vi "WS2812 Controller.vi"() -> ()   [LabVIEW 2017]
uses:
  IMAQCV/PIIO/Core/PIIO DIO.ctl
  IMAQCV/PIIO.lvlib
panel:
  in  "PIN":T1 items=["L1", "L2"]
  out "size(s)":i32
  in  "Number of LEDs":u16=40
  in  "Red Phase Multiplier":dbl=10.0 caption="Phase"
  in  "Red Phase Offset":dbl=10.0 caption="Phase"
  in  "Green Phase Multiplier":dbl=10.0 caption="Phase"
  in  "Green Phase Offset":dbl=10.0 caption="Phase"
  in  "Blue Phase Multiplier":dbl=10.0 caption="Phase"
  in  "Blue Phase Offset":dbl=10.0 caption="Phase"
  in  "Red Intensity Multiplier":dbl=1.0 caption="Phase" min=0.0 max=1.0
  in  "Green Intensity Multiplier":dbl=1.0 caption="Phase" min=0.0 max=1.0
  in  "Blue Intensity Multiplier":dbl=1.0 caption="Phase" min=0.0 max=1.0
  in  "Red Waveform":enum16{"Sine", "Square", "Triangle", "Sawtooth"}(ring)
  in  "Green Waveform":enum16{"Sine", "Square", "Triangle", "Sawtooth"}(ring)
  in  "Blue Waveform":enum16{"Sine", "Square", "Triangle", "Sawtooth"}(ring)
  in  "Red Duty Cycle":dbl=1.0 caption="Phase" min=0.0 max=100.0
  in  "Green Duty Cycle":dbl=1.0 caption="Phase" min=0.0 max=50.0
  in  "Blue Duty Cycle":dbl=1.0 caption="Phase" min=0.0 max=100.0
  in  "Stop Button":bool
  out "RGB Values":dynamicdata(graph)
  # "Duty Cycle\n(Square Wave)"
  # "Intensity (0-1)"
  # "Phase Multiplier"
  # "Phase Offset"
  # "Waveform"
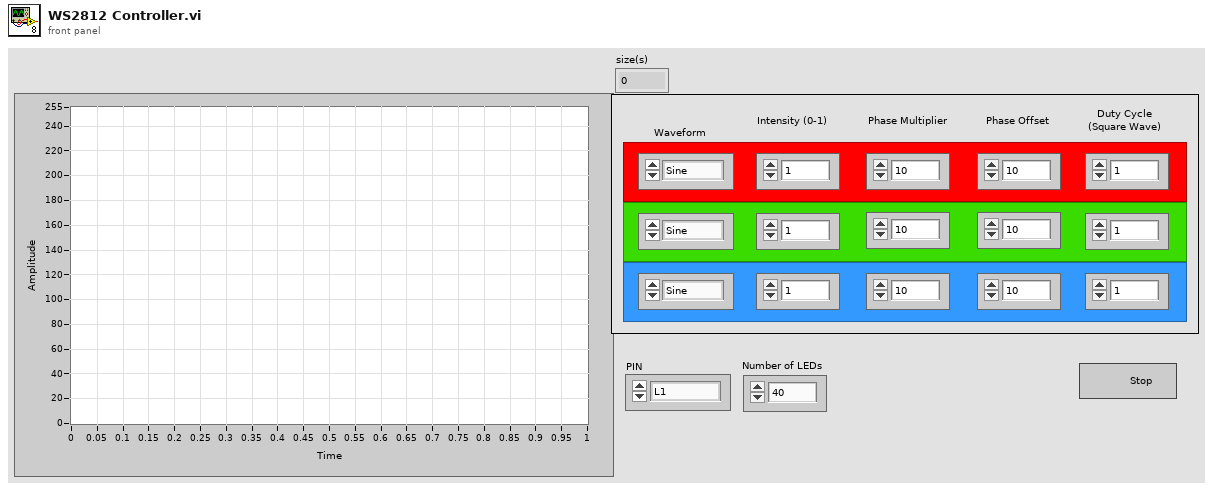
[diagram p1: front panel]
types:
  T1 = typedef "PIIO.lvlib/PIIO DIO.ctl" = u8
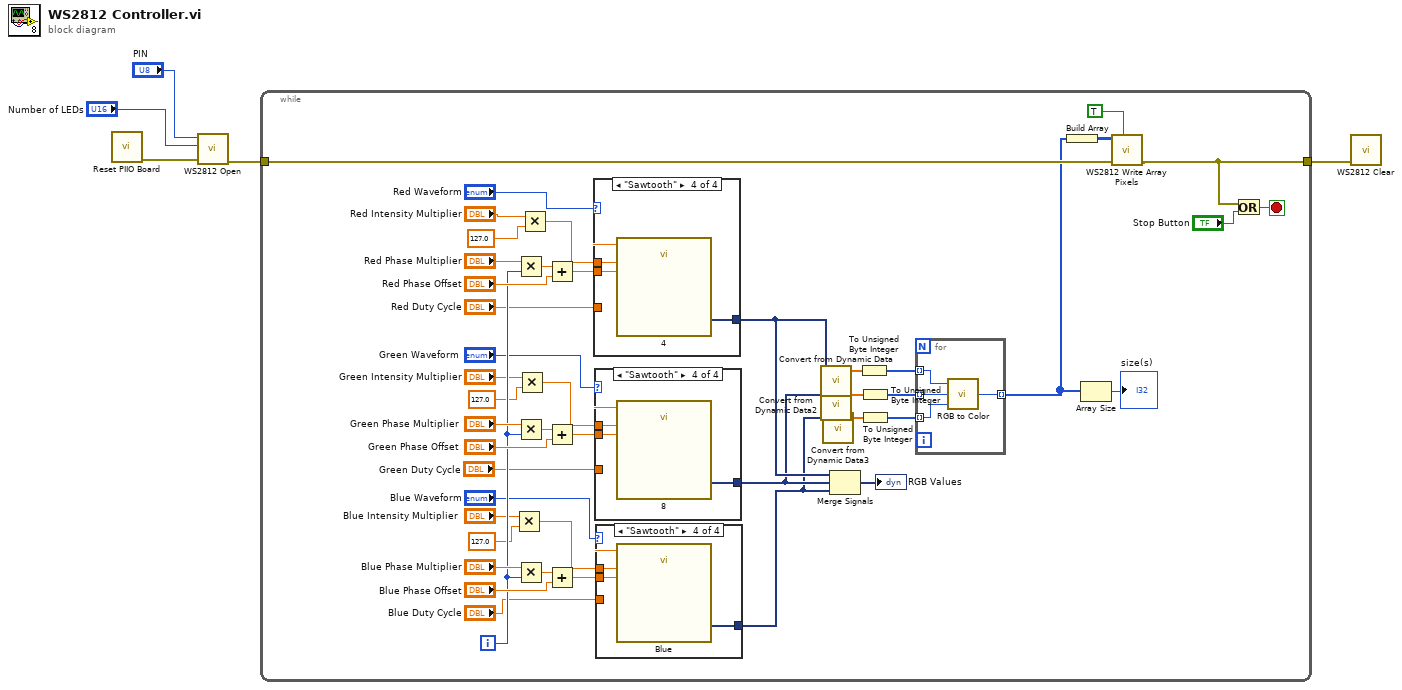
[diagram p0: block diagram]
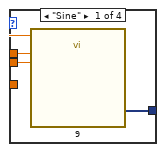
[diagram p2: hidden frame]
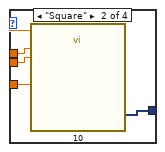
[diagram p3: hidden frame]
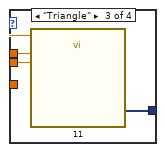
[diagram p4: hidden frame]
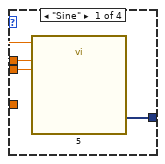
[diagram p5: hidden frame]
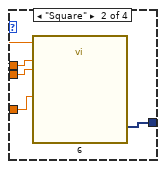
[diagram p6: hidden frame]
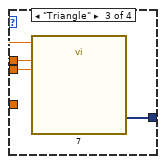
[diagram p7: hidden frame]
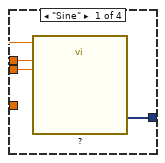
[diagram p8: hidden frame]
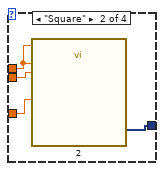
[diagram p9: hidden frame]
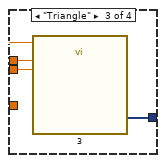
[diagram p10: hidden frame]
diagram:
  n1 = call "Reset PIIO Board.vi"() -> ("error out"=w2:errorcluster)  [unwired: 11 in]
  n2 = call "WS2812 Open.vi"("Error In"=w2, "Number of LEDs"="Number of LEDs", "PIN"="PIN") -> ("Error Out"=w5:errorcluster)  [unwired: 8 in]
  n3 = while {
    tunnel: w5 -> [w11]
    tunnel: [w10] -> w3
    i -> [w29]
    stop <- w51 stop-if-true
    n4 = Multiply(x="Blue Intensity Multiplier", y=127.0) -> (x*y=w19:dbl)
    n5 = Multiply(x="Red Phase Multiplier", y=w29) -> (x*y=w27:dbl)
    n6 = Multiply(x="Green Phase Multiplier", y=w29) -> (x*y=w45:dbl)
    n7 = Multiply(x="Blue Phase Multiplier", y=w29) -> (x*y=w42:dbl)
    n8 = Multiply(x="Green Intensity Multiplier", y=127.0) -> (x*y=w21:dbl)
    n9 = Multiply(x="Red Intensity Multiplier", y=127.0) -> (x*y=w20:dbl)
    n10 = Add(x=w27, y="Red Phase Offset") -> (x+y=w48:dbl)
    n11 = Add(x=w45, y="Green Phase Offset") -> (x+y=w47:dbl)
    n12 = Add(x=w42, y="Blue Phase Offset") -> (x+y=w40:dbl)
    n13 = case shown="\"Sawtooth\"" "Red Waveform" {
      tunnel: w48 -> [w80 w84 w87 w90]
      tunnel: [w79 w83 w86 w89] -> w33
      tunnel: w20 -> [w78 w82 w85 w88]
      tunnel: "Red Duty Cycle" -> [_ w81 _ _]
      frame "Sine" {
        n14 = call "?"("Offset"=w78, "Amplitude"=w78, "Phase"=w80) -> ("Red Sine"=w79:dynamicdata)  [unwired: 11 in, 1 out]
      }
      frame "Square" {
        n15 = call "2"("Offset"=w82, "Duty Cycle (%)"=w81, "Amplitude"=w82, "Phase"=w84) -> ("Red Square"=w83:dynamicdata)  [unwired: 10 in, 1 out]
      }
      frame "Triangle" {
        n16 = call "3"("Offset"=w85, "Amplitude"=w85, "Phase"=w87) -> ("Red Triangle"=w86:dynamicdata)  [unwired: 11 in, 1 out]
      }
      frame "Sawtooth" {
        n17 = call "4"("Offset"=w88, "Amplitude"=w88, "Phase"=w90) -> ("Red Sawtooth"=w89:dynamicdata)  [unwired: 11 in, 1 out]
      }
    }
    n18 = case shown="\"Sawtooth\"" "Green Waveform" {
      tunnel: w47 -> [w67 w71 w74 w77]
      tunnel: [w66 w70 w73 w76] -> w32
      tunnel: w21 -> [w65 w69 w72 w75]
      tunnel: "Green Duty Cycle" -> [_ w68 _ _]
      frame "Sine" {
        n19 = call "5"("Offset"=w65, "Amplitude"=w65, "Phase"=w67) -> ("Green Sine"=w66:dynamicdata)  [unwired: 11 in, 1 out]
      }
      frame "Square" {
        n20 = call "6"("Offset"=w69, "Duty Cycle (%)"=w68, "Amplitude"=w69, "Phase"=w71) -> ("Green Square"=w70:dynamicdata)  [unwired: 10 in, 1 out]
      }
      frame "Triangle" {
        n21 = call "7"("Offset"=w72, "Amplitude"=w72, "Phase"=w74) -> ("Green Triange"=w73:dynamicdata)  [unwired: 11 in, 1 out]
      }
      frame "Sawtooth" {
        n22 = call "8"("Offset"=w75, "Amplitude"=w75, "Phase"=w77) -> ("Green Sawtooth"=w76:dynamicdata)  [unwired: 11 in, 1 out]
      }
    }
    n23 = case shown="\"Sawtooth\"" "Blue Waveform" {
      tunnel: w40 -> [w54 w58 w61 w64]
      tunnel: [w53 w57 w60 w63] -> w31
      tunnel: w19 -> [w52 w56 w59 w62]
      tunnel: "Blue Duty Cycle" -> [_ w55 _ _]
      frame "Sine" {
        n24 = call "9"("Offset"=w52, "Amplitude"=w52, "Phase"=w54) -> ("Blue Sine"=w53:dynamicdata)  [unwired: 11 in, 1 out]
      }
      frame "Square" {
        n25 = call "10"("Offset"=w56, "Duty Cycle (%)"=w55, "Amplitude"=w56, "Phase"=w58) -> ("Blue Square"=w57:dynamicdata)  [unwired: 10 in, 1 out]
      }
      frame "Triangle" {
        n26 = call "11"("Offset"=w59, "Amplitude"=w59, "Phase"=w61) -> ("Blue Triangle"=w60:dynamicdata)  [unwired: 11 in, 1 out]
      }
      frame "Sawtooth" {
        n27 = call "Blue"("Offset"=w62, "Amplitude"=w62, "Phase"=w64) -> ("Blue Sawtooth"=w63:dynamicdata)  [unwired: 11 in, 1 out]
      }
    }
    n28 = call "Convert from Dynamic Data"("Dynamic Data Type"=w33) -> ("Array"=w39:dbl[])  [unwired: 3 in]
    n29 = call "Convert from Dynamic Data2"("Dynamic Data Type"=w32) -> ("Array"=w37:dbl[])  [unwired: 3 in]
    n30 = call "Convert from Dynamic Data3"("Dynamic Data Type"=w31) -> ("Array"=w34:dbl[])  [unwired: 3 in]
    n31 = Merge Signals(w33, w32, w31) -> (→"RGB Values":dynamicdata)
    n32 = To Unsigned Byte Integer(number=w39) -> (unsigned 8bit integer=w38:u8[])
    n33 = To Unsigned Byte Integer(number=w37) -> (unsigned 8bit integer=w36:u8[])
    n34 = To Unsigned Byte Integer(number=w34) -> (unsigned 8bit integer=w35:u8[])
    n35 = for {
      tunnel: w38 -> [w94] mode=indexing
      tunnel: [w93] -> w7 mode=indexing
      tunnel: w36 -> [w92] mode=indexing
      tunnel: w35 -> [w91] mode=indexing
      n36 = call <vilib>:"RGB to Color.vi"("B"=w91, "G"=w92, "R"=w94) -> ("Color"=w93:u32)
    }
    n37 = Build Array(w7) -> (w9:u32[][])
    n38 = Array Size(array=w7) -> (size(s)=→"size(s)":i32)
    n39 = call "WS2812 Write Array Pixels.vi"("Refresh? (True)"=TRUE, "Error In"=w11, "pixmap"=w9) -> ("Error Out"=w10:errorcluster)  [unwired: 8 in]
    n40 = Or(x=w10, y="Stop Button") -> (x .or. y?=w51:bool)
  }
  n41 = call "WS2812 Clear.vi"("Error In"=w3) -> ()  [unwired: 10 in, 1 out]
